vi "Calculate-temperature-field.vi"(8 "error in":errorcluster, 9 "Temp. params. ref. in":refnum<data-value>, 10 "Buffer element in":T1 {"Temperature characteristics"."Stand. dev. temperature" format="%#.1f"; "Temperature characteristics"."Min. temperature" format="%#.0f"; "Temperature characteristics"."Max. temperature" format="%#.0f"; "Temperature characteristics"."Average temperature" format="%#.0f"}) -> (0 "error IO":errorcluster, 1 "Temp. params. ref.":refnum<data-value>, 2 "Buffer element":T1 {"Temperature characteristics"."Stand. dev. temperature" format="%#.1f"; "Temperature characteristics"."Min. temperature" format="%#.0f"; "Temperature characteristics"."Max. temperature" format="%#.0f"; "Temperature characteristics"."Average temperature" format="%#.0f"})   [LabVIEW 2013, in "CameraVision.lvlib" / "CV-Temperature.lvclass"]
uses:
  CV-Temperature.lvclass
  Buffers/Storage-buffer.ctl
  <vilib>/vision/Image Controls.llb/IMAQ Image.ctl
  Temperature-characteristics.ctl
  Analysis/Characteristics-cluster.ctl
  CV-Temperature.lvclass/CV-Temperature.ctl
  Read TemperatureFieldRegression.vi
  Analysis/CV-Analysis.lvclass
  Buffers/CV-Buffers.lvclass
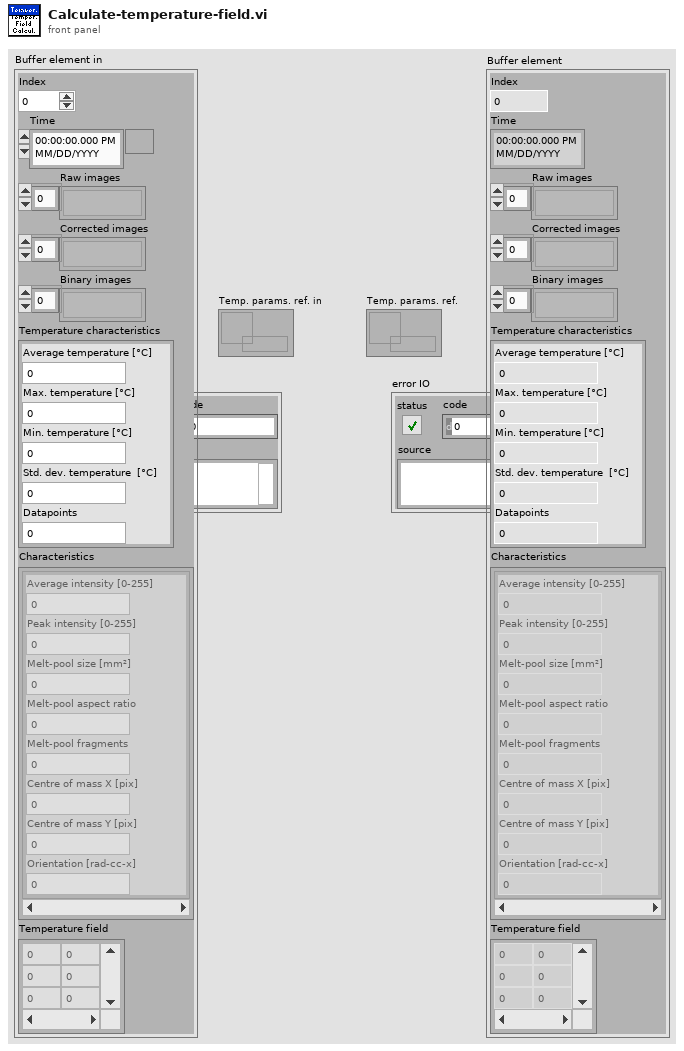
[diagram p1: front panel]
types:
  T1 = typedef "CameraVision.lvlib/CV-Buffers.lvclass/Storage-buffer.ctl" = cluster{"Index":i32, "Time":timestamp, "Raw images":T2[], "Corrected images":T2[], "Binary images":T2[], "Temperature characteristics":T3, "Characteristics":T4[], "Temperature field":dbl[][]}
  T2 = typedef "IMAQ Image.ctl" = refnum<image>
  T3 = typedef "CameraVision.lvlib/CV-Temperature.lvclass/Temperature-characteristics.ctl" = cluster{"Average temperature ":dbl, "Max. temperature":dbl, "Min. temperature":dbl, "Stand. dev. temperature":dbl, "Datapoints":dbl}
  T4 = typedef "CameraVision.lvlib/CV-Analysis.lvclass/Characteristics-cluster.ctl" = cluster{"Average intensity":dbl, "Peak intensity":dbl, "Melt-pool size":dbl, "Melt-pool aspect ratio":dbl, "Melt-pool fragments":dbl, "Centre of mass X":dbl, "Centre of mass Y":dbl, "Orientation":dbl}
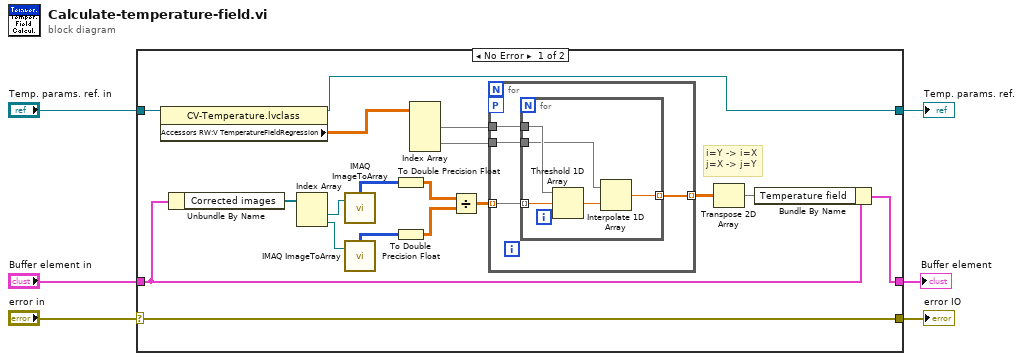
[diagram p0: block diagram]
diagram:
  n1 = case shown="No Error" "error in" {
    selector: "error in" -> [w17 w36]
    tunnel: [w17 w36] -> w6
    tunnel: "Temp. params. ref. in" -> [w20 w34]
    tunnel: "Buffer element in" -> [w8 w35]
    tunnel: [w18 w34] -> w2
    tunnel: [w7 w35] -> w1
    frame No Error {
      # "i=Y -> i=X\nj=X -> j=Y"
      n2 = property class="CV-Temperature.lvclass"(reference=w20) -> (reference out=w18:refnum<data-value>, "Accessors RW:V TemperatureFieldRegression"=w19:dbl[][])  [unwired: 1 in, 1 out]
      n3 = Unbundle By Name(w8) -> ("Corrected images"=w16:T2[])
      n4 = Index Array(array=w16) -> (element #1=w15:T2, element #2=w14:T2)  [unwired: 2 in]
      n5 = call "IMAQ ImageToArray"("Image"=w15) -> ("Image Pixels (U8)"=w11:u8[][])  [unwired: 3 in, 4 out]
      n6 = call "IMAQ ImageToArray"("Image"=w14) -> ("Image Pixels (U8)"=w13:u8[][])  [unwired: 3 in, 4 out]
      n7 = To Double Precision Float(number=w11) -> (double precision float=w10:dbl[][])
      n8 = To Double Precision Float(number=w13) -> (double precision float=w12:dbl[][])
      n9 = Index Array(array=w19) -> (element #1=w22:dbl[], element #2=w24:dbl[])  [unwired: 4 in]
      n10 = Divide(x=w10, y=w12) -> (x/y=w21:dbl[][])
      n11 = for {
        tunnel: w21 -> [w28] mode=indexing
        tunnel: w22 -> [w27]
        tunnel: w24 -> [w26]
        tunnel: [w25] -> w23 mode=indexing
        workers-P: _ -> [_]
        n12 = for {
          tunnel: w28 -> [w29] mode=indexing
          tunnel: w27 -> [w31]
          tunnel: w26 -> [w30]
          tunnel: [w32] -> w25 mode=indexing
          n13 = Threshold 1D Array(2:w29, 3:w31) -> (0:w33:dbl)  [unwired: 1 in]
          n14 = Interpolate 1D Array(1:w33, 2:w30) -> (0:w32:dbl)
        }
      }
      n15 = Transpose 2D Array(2D array=w23) -> (transposed array=w9:dbl[][])
      n16 = Bundle By Name(cluster=w8, "Temperature field"=w9) -> (w7:T1)
    }
    frame Error {
    }
  }
  "error IO" <- w6
  "Temp. params. ref." <- w2
  "Buffer element" <- w1
